vi "main - Copy.vi"() -> ()   [LabVIEW 2013]
uses:
  DB/ConfDB.ctl
  DB/ConfEnum.ctl
  DB/DbEnum.ctl
panel:
  out "Image Out":T1(plugin-control)
  in  "N times sigam (tol)":i32=5
  in  "Number of images to save around freeze point":i32=10
  in  "Number of Images":i32=100
  in  "File Path":path=path "Z:/Downloads/Fridge Pictures/1"
  out "Number of Matches":i32=25
  out "Matches (pixel)":T2(array[cluster])=[{"Position"={"x"=1341.5, "y"=734.5}, "Angle"=0.0, "Scale"=1.0, "Score"=1000.0, "Bounding Box"=[{"x"=1296.0, "y"=694.0}, {"x"=1387.0, "y"=694.0}, {"x"=1387.0, "y"=775.0}, {"x"=1296.0, "y"=775.0}, {"x"=1296.0, "y"=694.0}]}, {"Position"={"x"=1196.5743, "y"=1126.0432}, "Angle"=0.0, "Scale"=1.0, "Score"=900.23456, "Bounding Box"=[{"x"=1151.0743, "y"=1085.5432}, {"x"=1242.0743, "y"=1085.5432}, {"x"=1242.0743, "y"=1166.5432}, {"x"=1151.0743, "y"=1166.5432}, {"x"=1151.0743, "y"=1085.5432}]}, {"Position"={"x"=1545.7823, "y"=532.04376}, "Angle"=0.0, "Scale"=1.0, "Score"=892.0734, "Bounding Box"=[{"x"=1500.2823, "y"=491.54376}, {"x"=1591.2823, "y"=491.54376}, {"x"=1591.2823, "y"=572.54376}, {"x"=1500.2823, "y"=572.54376}, {"x"=1500.2823, "y"=491.54376}]}, {"Position"={"x"=1094.883, "y"=753.2342}, "Angle"=0.0, "Scale"=1.0, "Score"=891.1741, "Bounding Box"=[{"x"=1049.383, "y"=712.7342}, {"x"=1140.383, "y"=712.7342}, {"x"=1140.383, "y"=793.7342}, {"x"=1049.383, "y"=793.7342}, {"x"=1049.383, "y"=712.7342}]}, {"Position"={"x"=1371.3896, "y"=961.625}, "Angle"=0.0, "Scale"=1.0, "Score"=878.96686, "Bounding Box"=[{"x"=1325.8896, "y"=921.125}, {"x"=1416.8896, "y"=921.125}, {"x"=1416.8896, "y"=1002.125}, {"x"=1325.8896, "y"=1002.125}, {"x"=1325.8896, "y"=921.125}]}, {"Position"={"x"=1686.145, "y"=812.43805}, "Angle"=0.0, "Scale"=1.0, "Score"=825.67773, "Bounding Box"=[{"x"=1640.645, "y"=771.93805}, {"x"=1731.645, "y"=771.93805}, {"x"=1731.645, "y"=852.93805}, {"x"=1640.645, "y"=852.93805}, {"x"=1640.645, "y"=771.93805}]}, {"Position"={"x"=936.9166, "y"=624.4227}, "Angle"=0.0, "Scale"=1.0, "Score"=817.7966, "Bounding Box"=[{"x"=891.4166, "y"=583.9227}, {"x"=982.4166, "y"=583.9227}, {"x"=982.4166, "y"=664.9227}, {"x"=891.4166, "y"=664.9227}, {"x"=891.4166, "y"=583.9227}]}, {"Position"={"x"=1536.802, "y"=1190.3126}, "Angle"=0.0, "Scale"=1.0, "Score"=786.6126, "Bounding Box"=[{"x"=1491.302, "y"=1149.8126}, {"x"=1582.302, "y"=1149.8126}, {"x"=1582.302, "y"=1230.8126}, {"x"=1491.302, "y"=1230.8126}, {"x"=1491.302, "y"=1149.8126}]}, {"Position"={"x"=1679.4249, "y"=1001.6944}, "Angle"=0.0, "Scale"=1.0, "Score"=784.3884, "Bounding Box"=[{"x"=1633.9249, "y"=961.1944}, {"x"=1724.9249, "y"=961.1944}, {"x"=1724.9249, "y"=1042.1943}, {"x"=1633.9249, "y"=1042.1943}, {"x"=1633.9249, "y"=961.1944}]}, {"Position"={"x"=1229.3533, "y"=500.3024}, "Angle"=0.0, "Scale"=1.0, "Score"=773.35645, "Bounding Box"=[{"x"=1183.8533, "y"=459.8024}, {"x"=1274.8533, "y"=459.8024}, {"x"=1274.8533, "y"=540.80237}, {"x"=1183.8533, "y"=540.80237}, {"x"=1183.8533, "y"=459.8024}]}, {"Position"={"x"=951.5936, "y"=1321.2926}, "Angle"=0.0, "Scale"=1.0, "Score"=751.618, "Bounding Box"=[{"x"=906.0936, "y"=1280.7926}, {"x"=997.0936, "y"=1280.7926}, {"x"=997.0936, "y"=1361.7926}, {"x"=906.0936, "y"=1361.7926}, {"x"=906.0936, "y"=1280.7926}]}, {"Position"={"x"=1773.0933, "y"=552.07654}, "Angle"=0.0, "Scale"=1.0, "Score"=723.29376, "Bounding Box"=[{"x"=1727.5933, "y"=511.57654}, {"x"=1818.5933, "y"=511.57654}, {"x"=1818.5933, "y"=592.57654}, {"x"=1727.5933, "y"=592.57654}, {"x"=1727.5933, "y"=511.57654}]}, {"Position"={"x"=1248.5851, "y"=325.4367}, "Angle"=0.0, "Scale"=1.0, "Score"=719.0533, "Bounding Box"=[{"x"=1203.0851, "y"=284.9367}, {"x"=1294.0851, "y"=284.9367}, {"x"=1294.0851, "y"=365.9367}, {"x"=1203.0851, "y"=365.9367}, {"x"=1203.0851, "y"=284.9367}]}, {"Position"={"x"=1253.8042, "y"=1431.3312}, "Angle"=0.0, "Scale"=1.0, "Score"=717.0521, "Bounding Box"=[{"x"=1208.3042, "y"=1390.8312}, {"x"=1299.3042, "y"=1390.8312}, {"x"=1299.3042, "y"=1471.8312}, {"x"=1208.3042, "y"=1471.8312}, {"x"=1208.3042, "y"=1390.8312}]}, {"Position"={"x"=1508.0845, "y"=1397.7313}, "Angle"=0.0, "Scale"=1.0, "Score"=702.3233, "Bounding Box"=[{"x"=1462.5845, "y"=1357.2313}, {"x"=1553.5845, "y"=1357.2313}, {"x"=1553.5845, "y"=1438.2313}, {"x"=1462.5845, "y"=1438.2313}, {"x"=1462.5845, "y"=1357.2313}]}, {"Position"={"x"=1552.1433, "y"=304.62778}, "Angle"=0.0, "Scale"=1.0, "Score"=694.1083, "Bounding Box"=[{"x"=1506.6433, "y"=264.12778}, {"x"=1597.6433, "y"=264.12778}, {"x"=1597.6433, "y"=345.12778}, {"x"=1506.6433, "y"=345.12778}, {"x"=1506.6433, "y"=264.12778}]}, {"Position"={"x"=786.0882, "y"=1109.9098}, "Angle"=0.0, "Scale"=1.0, "Score"=691.0762, "Bounding Box"=[{"x"=740.5882, "y"=1069.4098}, {"x"=831.5882, "y"=1069.4098}, {"x"=831.5882, "y"=1150.4098}, {"x"=740.5882, "y"=1150.4098}, {"x"=740.5882, "y"=1069.4098}]}, {"Position"={"x"=1926.0133, "y"=864.04224}, "Angle"=0.0, "Scale"=1.0, "Score"=639.03375, "Bounding Box"=[{"x"=1880.5133, "y"=823.54224}, {"x"=1971.5133, "y"=823.54224}, {"x"=1971.5133, "y"=904.54224}, {"x"=1880.5133, "y"=904.54224}, {"x"=1880.5133, "y"=823.54224}]}, {"Position"={"x"=1927.5698, "y"=665.46716}, "Angle"=0.0, "Scale"=1.0, "Score"=624.3622, "Bounding Box"=[{"x"=1882.0698, "y"=624.96716}, {"x"=1973.0698, "y"=624.96716}, {"x"=1973.0698, "y"=705.96716}, {"x"=1882.0698, "y"=705.96716}, {"x"=1882.0698, "y"=624.96716}]}, {"Position"={"x"=1036.6719, "y"=924.2498}, "Angle"=0.0, "Scale"=1.0, "Score"=622.71356, "Bounding Box"=[{"x"=991.1719, "y"=883.7498}, {"x"=1082.1719, "y"=883.7498}, {"x"=1082.1719, "y"=964.7498}, {"x"=991.1719, "y"=964.7498}, {"x"=991.1719, "y"=883.7498}]}, {"Position"={"x"=1798.4291, "y"=427.18503}, "Angle"=0.0, "Scale"=1.0, "Score"=612.04645, "Bounding Box"=[{"x"=1752.9291, "y"=386.68503}, {"x"=1843.9291, "y"=386.68503}, {"x"=1843.9291, "y"=467.68503}, {"x"=1752.9291, "y"=467.68503}, {"x"=1752.9291, "y"=386.68503}]}, {"Position"={"x"=679.48035, "y"=781.2287}, "Angle"=0.0, "Scale"=1.0, "Score"=604.38666, "Bounding Box"=[{"x"=633.98035, "y"=740.7287}, {"x"=724.98035, "y"=740.7287}, {"x"=724.98035, "y"=821.7287}, {"x"=633.98035, "y"=821.7287}, {"x"=633.98035, "y"=740.7287}]}, {"Position"={"x"=1858.5896, "y"=1175.5317}, "Angle"=0.0, "Scale"=1.0, "Score"=601.6367, "Bounding Box"=[{"x"=1813.0896, "y"=1135.0317}, {"x"=1904.0896, "y"=1135.0317}, {"x"=1904.0896, "y"=1216.0317}, {"x"=1813.0896, "y"=1216.0317}, {"x"=1813.0896, "y"=1135.0317}]}, {"Position"={"x"=873.6445, "y"=427.1809}, "Angle"=0.0, "Scale"=1.0, "Score"=584.28125, "Bounding Box"=[{"x"=828.1445, "y"=386.6809}, {"x"=919.1445, "y"=386.6809}, {"x"=919.1445, "y"=467.6809}, {"x"=828.1445, "y"=467.6809}, {"x"=828.1445, "y"=386.6809}]}, {"Position"={"x"=599.6848, "y"=551.81195}, "Angle"=0.0, "Scale"=1.0, "Score"=543.92706, "Bounding Box"=[{"x"=554.1848, "y"=511.31195}, {"x"=645.1848, "y"=511.31195}, {"x"=645.1848, "y"=592.31195}, {"x"=554.1848, "y"=592.31195}, {"x"=554.1848, "y"=511.31195}]}]
  in  "Start Index":i32=1
  in  "File Name":string="cameraA-nr"
  out "error out":errorcluster
  in  "error in":errorcluster
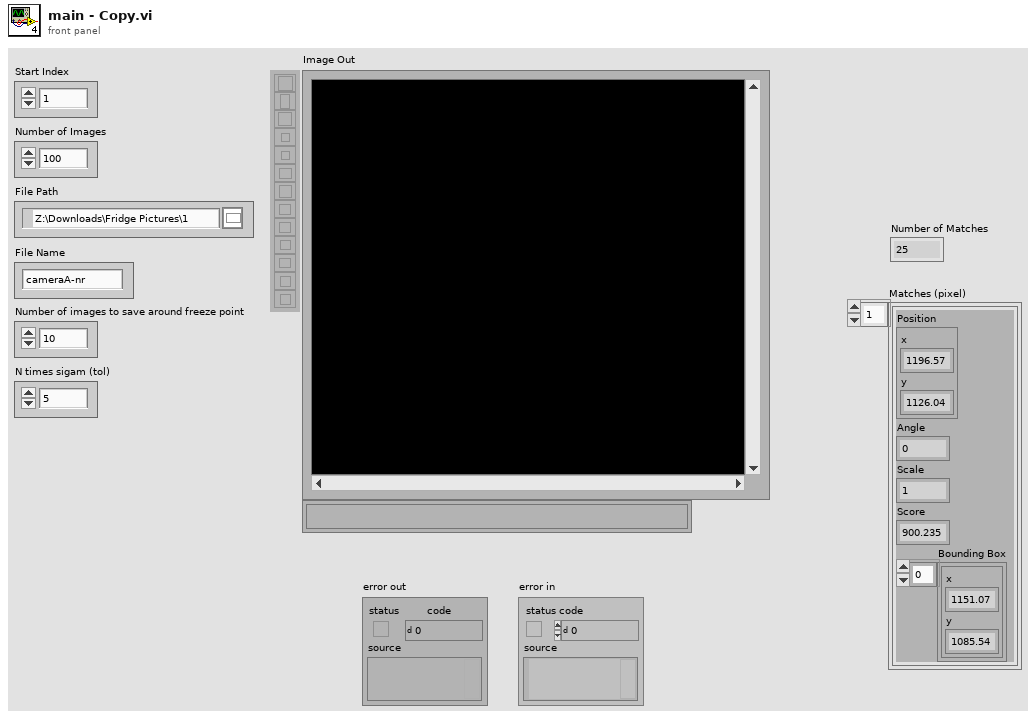
[diagram p1: front panel]
types:
  T1 = typedef "IMAQ Image.ctl" = refnum<image>
  T2 = cluster{"Position":cluster{"x":sgl, "y":sgl}, "Angle":sgl, "Scale":sgl, "Score":sgl, "Bounding Box":cluster{"x":sgl, "y":sgl}[]}[]
  T3 = typedef "DbEnum.ctl" = enum16{"Init", "Insert Detection Result Data", "GetDropletsBoundingBox"}
  T4 = typedef "ConfEnum.ctl" = enum16{"Init", "Configure DB"}
  T5 = typedef "ConfDB.ctl" = cluster{"NumberOfImages":i32, "NoImages2SaveAroundFreeze":i32, "Path":path, "NameOfPartialFile":string, "StartIndex":i32, "NumberOfStdTol":i32}
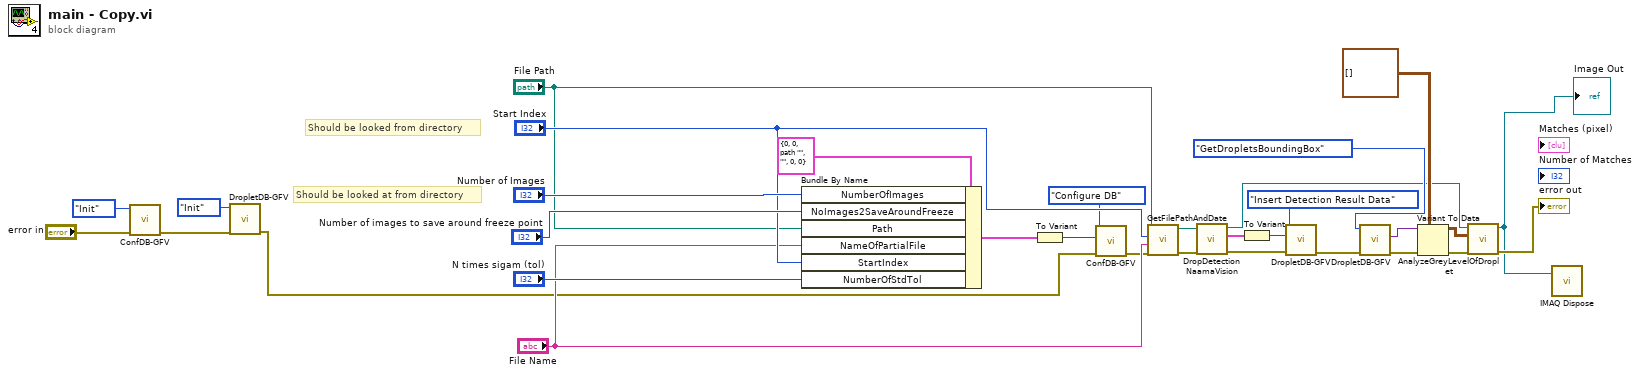
[diagram p0: block diagram]
diagram:
  # "Should be looked from directory"
  # "Should be looked at from directory"
  n1 = call "ConfDB-GFV.vi"("error in (no error)"="error in", "Command In"=ConfEnum."Init" ("Command")) -> ("error out"=w13:errorcluster)  [unwired: 8 in, 1 out]
  n2 = call "DropletDB-GFV.vi"("error in (no error)"=w13, "Command In"=DbEnum."Init") -> ("error out"=w20:errorcluster)  [unwired: 8 in, 1 out]
  n3 = Bundle By Name(cluster=T5 {"NumberOfImages"=0, "NoImages2SaveAroundFreeze"=0, "Path"=path "", "NameOfPartialFile"="", "StartIndex"=0, "NumberOfStdTol"=0} ("ConfDB"), "NumberOfImages"="Number of Images", "NoImages2SaveAroundFreeze"="Number of images to save around freeze point", "Path"="File Path", "NameOfPartialFile"="File Name", "StartIndex"="Start Index", "NumberOfStdTol"="N times sigam (tol)") -> (w25:T5)
  n4 = To Variant(anything=w25) -> (Variant=w24:variant)
  n5 = call "ConfDB-GFV.vi"("error in (no error)"=w20, "Data in"=w24, "Command In"=ConfEnum."Configure DB") -> ("error out"=w23:errorcluster)  [unwired: 7 in, 1 out]
  n6 = call "GetFilePathAndDate.vi"("error in (no error)"=w23, "String"="File Name", "Index"="Start Index", "Path"="File Path") -> ("error out"=w16:errorcluster, "file out"=w32:path)  [unwired: 5 in, 1 out]
  n7 = call "DropDetection NaamaVision.vi"("error in"=w16, "Path"=w32) -> ("error out"=w15:errorcluster, "Matches (pixel)"=w19:T2, "Image Out"=w4:T1)  [unwired: 6 in, 1 out]
  n8 = To Variant(anything=w19) -> (Variant=w18:variant)
  n9 = call "DropletDB-GFV.vi"("error in (no error)"=w15, "Data in"=w18, "Command In"=DbEnum."Insert Detection Result Data") -> ("error out"=w10:errorcluster)  [unwired: 7 in, 1 out]
  n10 = call "DropletDB-GFV.vi"("error in (no error)"=w10, "Command In"=DbEnum."GetDropletsBoundingBox") -> ("error out"=w8:errorcluster, "Data out"=w7:variant)  [unwired: 8 in]
  n11 = Variant To Data(error in=w8, type=cluster{"x":sgl, "y":sgl}[][] [] ("Bounding Box"), Variant=w7) -> (data=w5:cluster{"x":sgl, "y":sgl}[][], error out=w3:errorcluster)
  n12 = call "AnalyzeGreyLevelOfDroplet.vi"("error in (no error)"=w3, "Bounding Box"=w5, "Image In"=w4) -> ("error out"=→"error out":errorcluster, "Image Out"=w1:T1)  [unwired: 7 in]
  "Image Out" <- w1
  n13 = call "IMAQ Dispose"("Image"=w1) -> ()  [unwired: 5 in, 1 out]
